vi "OntrakControll.vi"(1 "Channel\nto Set":u16(ring) items=["0", "1", "2", "3", "4", "5", "6", "7"], 2 "Set/Read":enum16{"Read Channel", "Set Channel"}(ring), 3 "Comport":refnum<visa-resource-name>="COM1") -> (0 "Channel Read":string)   [LabVIEW 2013]
uses:
  <vilib>/Instr/_visa.llb/VISA Configure Serial Port (Instr).vi
panel:
  in  "Tab Control":enum32{"Main", "Setup", "Error"}(tab)
  out "error":errorcluster
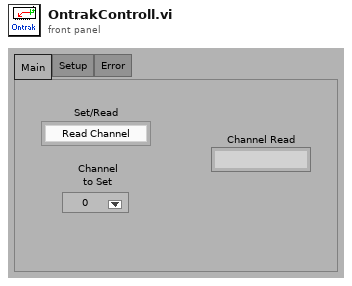
[diagram p1: front panel]
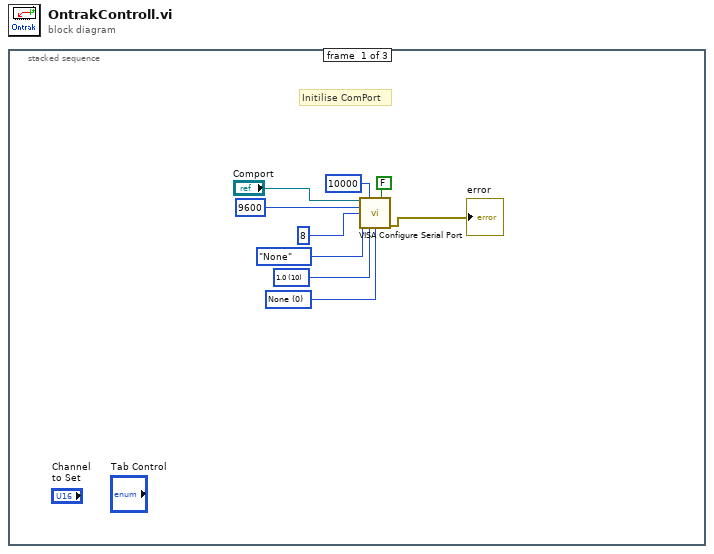
[diagram p0: block diagram]
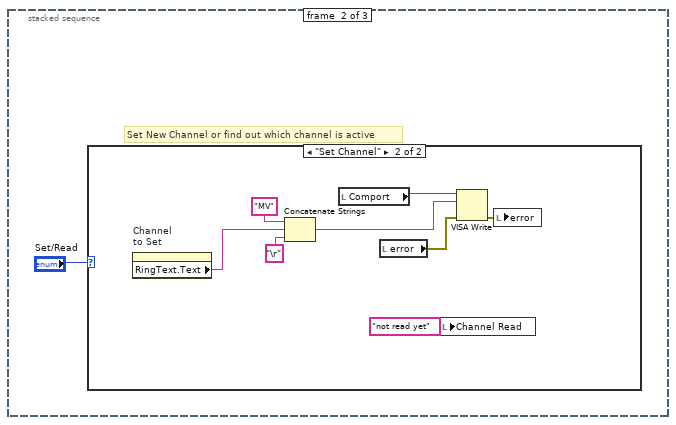
[diagram p2: hidden frame]
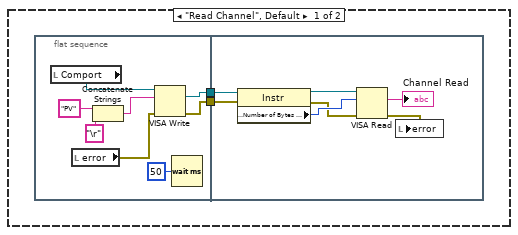
[diagram p3: hidden frame]
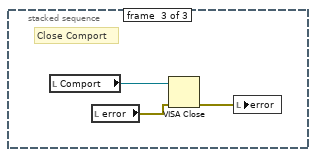
[diagram p4: hidden frame]
diagram:
  n1 = stacked-sequence {
    frame #0 {
      w2 = u16 10 items=["1.0"=10, "1.5"=15, "2.0"=20] ("stop bits (10: 1 bit)")
      w3 = u16 0 items=["None", "XON/XOFF", "RTS/CTS", "XON/XOFF & RTS/CTS", "DTR/DSR", "XON/XOFF & DTR/DSR"] ("flow control (0:none)")
      # "Initilise ComPort"
      n2 = call-poly "VISA Configure Serial Port"("VISA resource name"="Comport", "timeout (10sec)"=u32 10000, "Enable Termination\nChar (T)"=FALSE ("Enable Termination\nChar (T)"), "baud rate (9600)"=u32 9600, "data bits (8)"=u16 8, "parity (0:none)"=enum16{"None", "Odd", "Even", "Mark", "Space"}."None", "stop bits (10: 1 bit)"=w2, "flow control (0:none)"=w3) -> ("error out"=→"error":errorcluster)  [unwired: 1 in, 6 out]
    }
    frame #1 {
      # "Set New Channel or find out which channel is active"
      n3 = case shown="\"Set Channel\"" "Set/Read" {
        frame "Read Channel", Default {
          n4 = flat-sequence {
            tunnel: [w15] -> w12
            tunnel: [w14] -> w11
            tunnel: w12 -> [w22]
            tunnel: w11 -> [w21]
            frame #0 {
              n5 = local read "Comport"() -> (w20:refnum<visa-resource-name>)
              n6 = local read "error"() -> (w19:errorcluster)
              n7 = Concatenate Strings("PV" ("write buffer"), "\r") -> (w16:string)
              n8 = VISA Write(VISA resource name=w20, write buffer=w16, error in (no error)=w19) -> (VISA resource name out=w15:refnum<visa-resource-name>, error out=w14:errorcluster)  [unwired: 1 out]
              n9 = Wait (ms)(milliseconds to wait=u32 50) -> ()  [unwired: 1 out]
            }
            frame #1 {
              n10 = property class="Instr"(reference=w22, error in=w21) -> (reference out=w25:refnum<visa-resource-name>, error out=w23:errorcluster, "Serial Settings:Number of Bytes at Serial Port"=w24:u32)
              n11 = VISA Read(VISA resource name=w25, byte count=w24, error in (no error)=w23) -> (read buffer=→"Channel Read":string, error out=w27:errorcluster)  [unwired: 2 out]
              n12 = local write "error"(w27) -> ()
            }
          }
        }
        frame "Set Channel" {
          n13 = property on="Channel\nto Set" class="Ring (strict)"() -> ("RingText.Text"=w28:string)  [unwired: 2 in, 2 out]
          n14 = Concatenate Strings("MV", w28, "\r") -> (w31:string)
          n15 = local read "Comport"() -> (w35:refnum<visa-resource-name>)
          n16 = local read "error"() -> (w34:errorcluster)
          n17 = local write "Channel Read"("not read yet" ("Channel Read")) -> ()
          n18 = VISA Write(VISA resource name=w35, write buffer=w31, error in (no error)=w34) -> (error out=w30:errorcluster)  [unwired: 2 out]
          n19 = local write "error"(w30) -> ()
        }
      }
    }
    frame #2 {
      # "Close Comport"
      n20 = local read "Comport"() -> (w38:refnum<visa-resource-name>)
      n21 = local read "error"() -> (w36:errorcluster)
      n22 = VISA Close(VISA resource name=w38, error in (no error)=w36) -> (error out=w37:errorcluster)
      n23 = local write "error"(w37) -> ()
    }
  }
